vi "Close Read Reference.vi"(8 "error in":errorcluster, 11 "TDMS in":refnum<class "TDMS.lvclass">) -> (0 "error out":errorcluster, 3 "TDMS out":refnum<class "TDMS.lvclass">)   [LabVIEW 2019, in "TDMS.lvlib" / "TDMS.lvclass"]
uses:
  TDMS.lvclass
  TDMS.lvclass/TDMS.ctl
  Accessors/Read TDMS Read Ref.vi
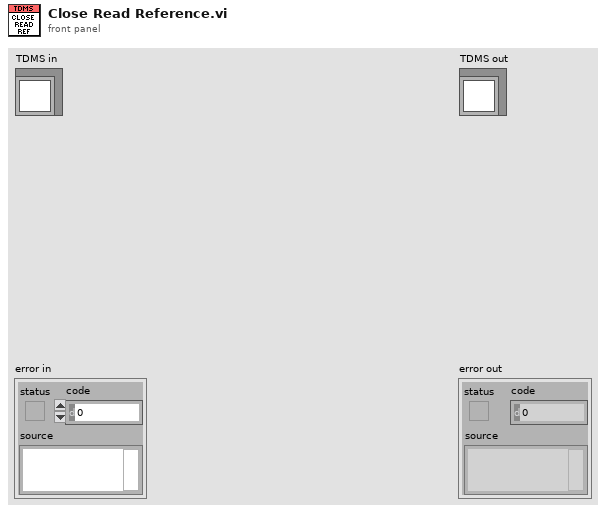
[diagram p1: front panel]
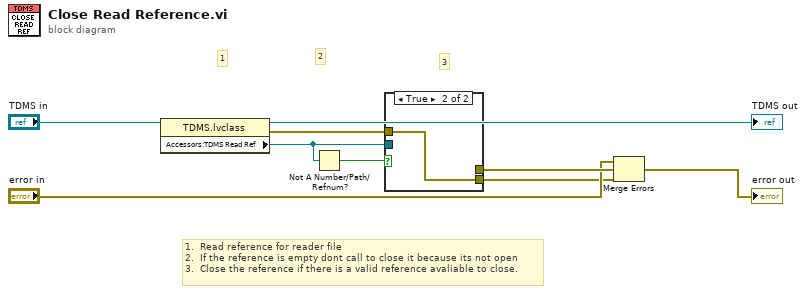
[diagram p0: block diagram]
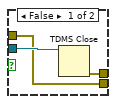
[diagram p2: hidden frame]
diagram:
  # "1.  Read reference for reader file\n2.  If the reference is empty dont call to close it because its not open\n3.  Close the reference if there is a valid reference avaliable to close."
  # "3"
  # "2"
  # "1"
  n1 = property class="TDMS.lvclass"(reference="TDMS in") -> (reference out=→"TDMS out":refnum<class "TDMS.lvclass">, error out=w3:errorcluster, "Accessors:TDMS Read Ref"=w1:refnum<k34>)  [unwired: 1 in]
  n2 = Not A Number/Path/Refnum?(number/path/refnum=w1) -> (NaN/Path/Refnum?=w4:bool)
  n3 = case shown="True" w4 {
    tunnel: [w12 _] -> w8
    tunnel: w1 -> [w11 _]
    tunnel: w3 -> [w10 w13]
    tunnel: [w10 w13] -> w2
    frame False {
      n4 = TDMS Close(11:w11) -> (0:w12:errorcluster)  [unwired: 1 in, 1 out]
    }
    frame True {
    }
  }
  n5 = Merge Errors("error in", w8, w2) -> (→"error out":errorcluster)
